vi "Sub_Set_Current_Measurement.vi"(0 "AgB29xxLib.IAgB29xx2":refnum<k7>, 5 "i":i32, 7 "AutoRangeEnabled":bool, 9 "NPLC":dbl=0.1, 11 "error in":errorcluster) -> (4 "AgB29xxLib.IAgB29xx2 2":refnum<k7>, 15 "error out":errorcluster)   [LabVIEW 2009]
panel:
  # "Sub VI: Set Current Measurement"
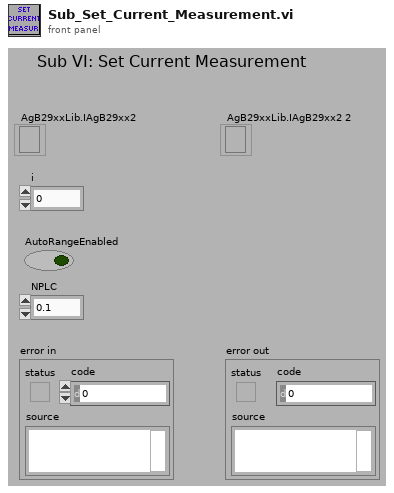
[diagram p1: front panel]
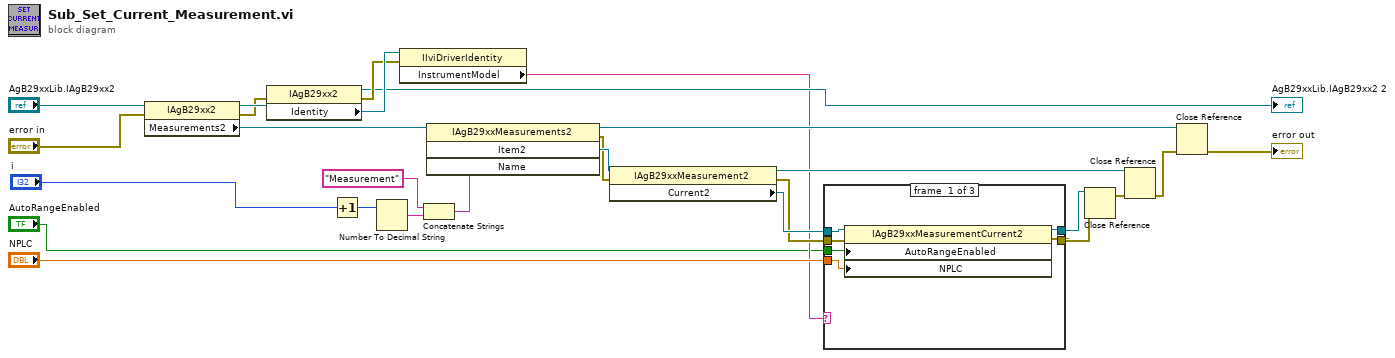
[diagram p0: block diagram]
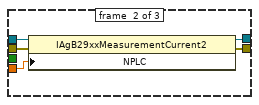
[diagram p2: hidden frame]
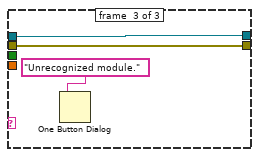
[diagram p3: hidden frame]
diagram:
  n1 = property class="IAgB29xx2"(reference="AgB29xxLib.IAgB29xx2", error in="error in") -> (reference out=w7:refnum<k7>, error out=w4:errorcluster, "Measurements2"=w24:refnum<k7>)
  n2 = property class="IAgB29xx2"(reference=w7, error in=w4) -> (reference out=→"AgB29xxLib.IAgB29xx2 2":refnum<k7>, error out=w5:errorcluster, "Identity"=w6:refnum<k7>)
  n3 = Increment(x="i") -> (x+1=w22:i32)
  n4 = Number To Decimal String(number=w22) -> (decimal integer string=w21:string)  [unwired: 1 in]
  n5 = property class="IIviDriverIdentity"(reference=w6, error in=w5) -> ("InstrumentModel"=w2:string)  [unwired: 2 out]
  n6 = Concatenate Strings("Measurement" ("string"), w21) -> (w19:string)
  n7 = invoke class="IAgB29xxMeasurements2" method="Item2"(reference=w24, "Name"=w19) -> (reference out=w14:refnum<k7>, error out=w18:errorcluster, "Item2"=w23:refnum<k7>)  [unwired: 2 in, 1 out]
  n8 = property class="IAgB29xxMeasurement2"(reference=w23, error in=w18) -> (reference out=w16:refnum<k7>, error out=w11:errorcluster, "Current2"=w12:refnum<k7>)
  n9 = case shown="\"B2961A\", \"B2962A\"" w2 {
    tunnel: [w33 w38 w40] -> w9
    tunnel: [w32 w37 w39] -> w8
    tunnel: w12 -> [w31 w35 w40]
    tunnel: w11 -> [w30 w36 w39]
    tunnel: "NPLC" -> [w28 w34 _]
    tunnel: "AutoRangeEnabled" -> [w29 _ _]
    frame #0 {
      n10 = property class="IAgB29xxMeasurementCurrent2"(reference=w31, error in=w30, "AutoRangeEnabled"=w29, "NPLC"=w28) -> (reference out=w33:refnum<k7>, error out=w32:errorcluster)
    }
    frame #1 {
      n11 = property class="IAgB29xxMeasurementCurrent2"(reference=w35, error in=w36, "NPLC"=w34) -> (reference out=w38:refnum<k7>, error out=w37:errorcluster)
    }
    frame #2 {
      n12 = One Button Dialog(message="Unrecognized module.") -> ()  [unwired: 1 in, 1 out]
    }
  }
  n13 = Close Reference(reference=w9, error in (no error)=w8) -> (error out=w17:errorcluster)
  n14 = Close Reference(reference=w16, error in (no error)=w17) -> (error out=w15:errorcluster)
  n15 = Close Reference(reference=w14, error in (no error)=w15) -> (error out=→"error out":errorcluster)
